vi "PointInAngleLine.vi"(4 "PointY":dbl(slide)=3.0 scale=-3.0..3.0, 6 "PointX":dbl(slide)=3.0 scale=-3.0..3.0, 7 "Angle (D: 10)":dbl=10.0, 8 "Line2Y":dbl, 9 "Line2X":dbl, 10 "Line1Y":dbl=2.0 format="%#_13g", 11 "Line1X":dbl=2.0 format="%#_13g") -> (2 "In Angle?":bool=TRUE)   [LabVIEW 2014]
panel:
  in  "milliseconds to wait":u32
  out "XY Graph":cluster{dbl[], dbl[]}[](graph)=[{[2.0, 0.0], [2.0, 0.0]}, {[3.0], [3.0]}]
  # "Forward"
  # "Back"
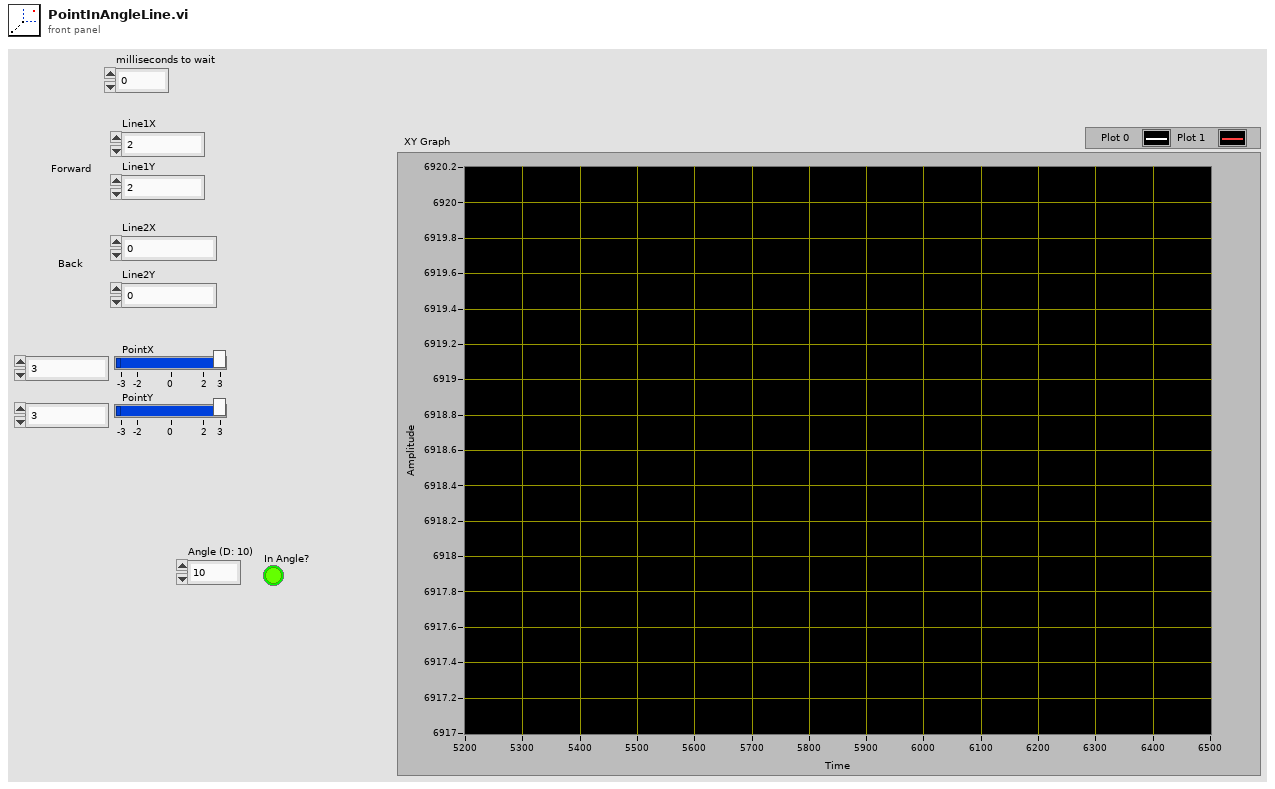
[diagram p1: front panel]
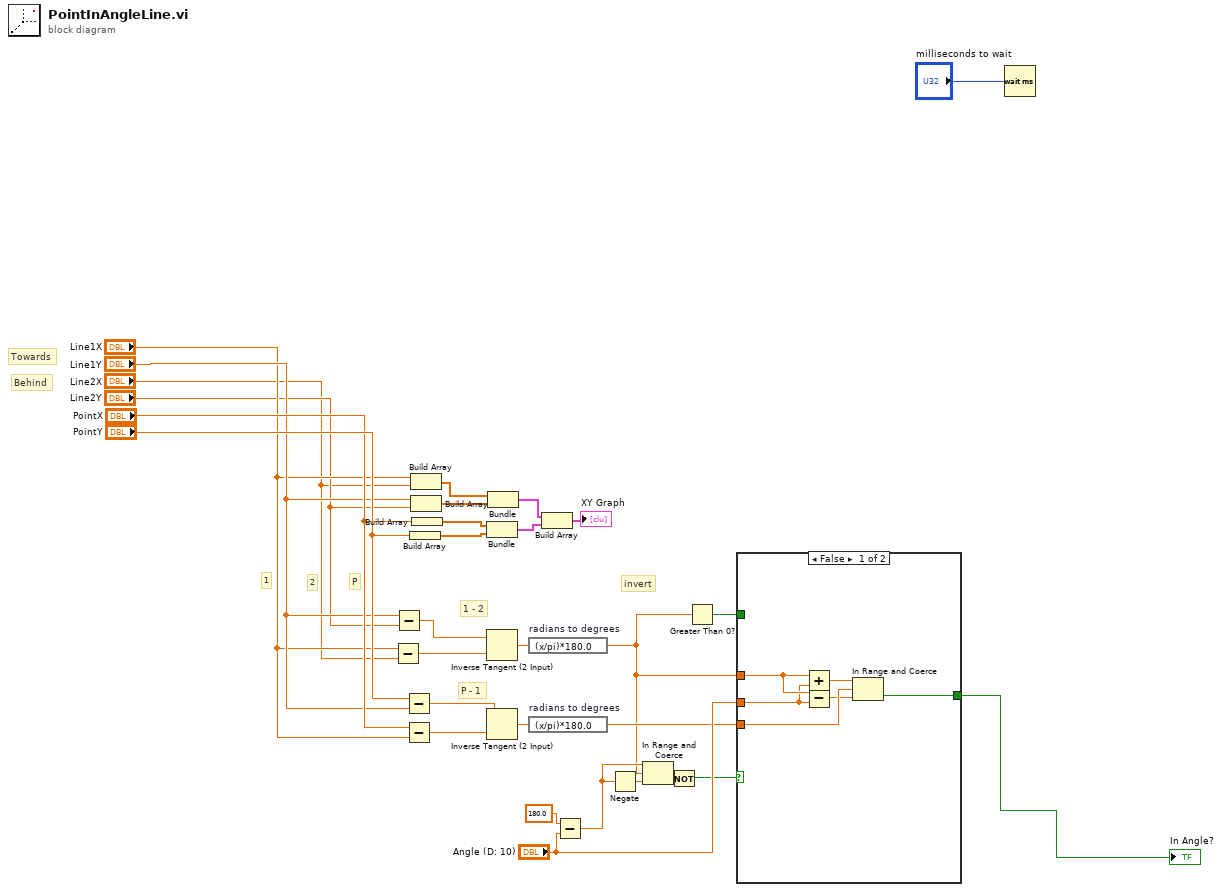
[diagram p0: block diagram]
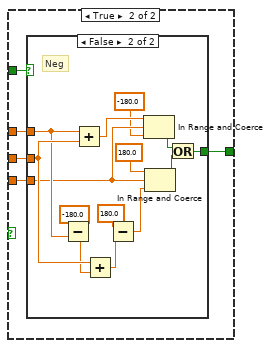
[diagram p2: hidden frame]
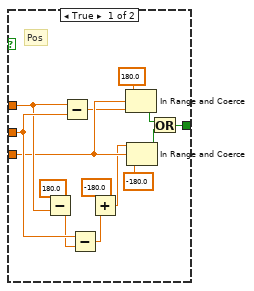
[diagram p3: hidden frame]
diagram:
  # "invert"
  # "Behind"
  # "Towards"
  # "P"
  # "2"
  # "1"
  # "1 - 2"
  # "P - 1"
  n1 = Subtract(x="Line1X", y="Line2X") -> (x-y=w18:dbl)
  n2 = Subtract(x="Line1Y", y="Line2Y") -> (x-y=w17:dbl)
  n3 = Subtract(x="PointY", y="Line1Y") -> (x-y=w15:dbl)
  n4 = Subtract(x="PointX", y="Line1X") -> (x-y=w16:dbl)
  n5 = Build Array("PointY") -> (w24:dbl[])
  n6 = Build Array("Line1X", "Line2X") -> (w27:dbl[])
  n7 = Build Array("Line1Y", "Line2Y") -> (w26:dbl[])
  n8 = Build Array("PointX") -> (w25:dbl[])
  n9 = Bundle(w25, w24) -> (w23:cluster{dbl[], dbl[]})  [unwired: 1 in]
  n10 = Inverse Tangent (2 Input)(1:w18, 2:w17) -> (0:w20:dbl)
  n11 = Inverse Tangent (2 Input)(1:w16, 2:w15) -> (0:w19:dbl)
  n12 = Bundle(w27, w26) -> (w22:cluster{dbl[], dbl[]})  [unwired: 1 in]
  n13 = expression code="(x/pi)*180.0" "radians to degrees"(w20) -> (w6:dbl)
  n14 = expression code="(x/pi)*180.0" "radians to degrees"(w19) -> (w8:dbl)
  n15 = Build Array(w22, w23) -> (→"XY Graph":cluster{dbl[], dbl[]}[])
  n16 = Subtract(x=180.0, y="Angle (D: 10)") -> (x-y=w12:dbl)
  n17 = Negate(x=w12) -> (-x=w13:dbl)
  n18 = In Range and Coerce(upper limit=w12, x=w6, lower limit=w13) -> (In Range?=w11:bool)  [unwired: 1 out]
  n19 = Not(x=w11) -> (.not. x?=w9:bool)
  n20 = Greater Than 0?(x=w6) -> (x > 0?=w7:bool)
  n21 = case shown="False" w9 {
    tunnel: w8 -> [w36 w38]
    tunnel: [w33 w40] -> w5
    tunnel: w6 -> [w32 w37]
    tunnel: "Angle (D: 10)" -> [w31 w39]
    tunnel: w7 -> [_ w41]
    frame False {
      n22 = Add(x=w32, y=w31) -> (x+y=w35:dbl)
      n23 = Subtract(x=w32, y=w31) -> (x-y=w34:dbl)
      n24 = In Range and Coerce(upper limit=w35, x=w36, lower limit=w34) -> (In Range?=w33:bool)  [unwired: 1 out]
    }
    frame True {
      n25 = case shown="False" w41 {
        tunnel: [w50 w64] -> w40
        tunnel: w39 -> [w54 w68]
        tunnel: w38 -> [w46 w60]
        tunnel: w37 -> [w47 w61]
        frame True {
          # "Pos"
          n26 = Subtract(x=180.0, y=w47) -> (x-y=w53:dbl)
          n27 = Subtract(x=w47, y=w54) -> (x-y=w45:dbl)
          n28 = Subtract(x=w54, y=w53) -> (x-y=w51:dbl)
          n29 = Add(x=-180.0, y=w51) -> (x+y=w43:dbl)
          n30 = In Range and Coerce(upper limit=180.0, x=w46, lower limit=w45) -> (In Range?=w48:bool)  [unwired: 1 out]
          n31 = In Range and Coerce(upper limit=w43, x=w46, lower limit=-180.0) -> (In Range?=w49:bool)  [unwired: 1 out]
          n32 = Or(x=w48, y=w49) -> (x .or. y?=w50:bool)
        }
        frame False {
          # "Neg"
          n33 = Subtract(x=-180.0, y=w61) -> (x-y=w67:dbl)
          n34 = Add(x=w61, y=w68) -> (x+y=w59:dbl)
          n35 = Add(x=w68, y=w67) -> (x+y=w65:dbl)
          n36 = Subtract(x=180.0, y=w65) -> (x-y=w57:dbl)
          n37 = In Range and Coerce(upper limit=w59, x=w60, lower limit=-180.0) -> (In Range?=w62:bool)  [unwired: 1 out]
          n38 = In Range and Coerce(upper limit=180.0, x=w60, lower limit=w57) -> (In Range?=w63:bool)  [unwired: 1 out]
          n39 = Or(x=w62, y=w63) -> (x .or. y?=w64:bool)
        }
      }
    }
  }
  "In Angle?" <- w5
  n40 = Wait (ms)(milliseconds to wait="milliseconds to wait") -> ()  [unwired: 1 out]
